vi "VRMQtest.vi"() -> ()   [LabVIEW 2019]
panel:
  out "read buffer":string
  in  "IP Address":string="172.16.136.21"
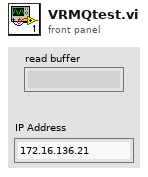
[diagram p1: front panel]
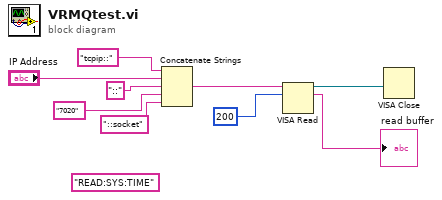
[diagram p0: block diagram]
diagram:
  (unwired) "READ:SYS:TIME" ("Command String")
  n1 = Concatenate Strings("tcpip::" ("string"), "IP Address", "::" ("string"), "7020" ("string"), "::socket" ("string")) -> (w1:string)
  n2 = VISA Read(VISA resource name=w1, byte count=u32 200) -> (VISA resource name out=w2:refnum<visa-resource-name>, read buffer=→"read buffer":string)  [unwired: 1 in, 2 out]
  n3 = VISA Close(VISA resource name=w2) -> ()  [unwired: 1 in, 1 out]
